vi "Load and Save Data (Burst Shape Data).vi"(0 "VISA resource name":refnum<visa-resource-name>, 1 "Rise Points Values":dbl[](array[numeric])=[0.0, 0.0] format="%.1f", 5 "Destination File":string, 7 "Rise Points(2)":u32=2, 9 "Fall Points(2)":u32=2, 11 "error in (no error)":errorcluster, 12 "Fall Points Values":dbl[](array[numeric])=[0.0, 0.0] format="%.1f") -> (4 "VISA resource name out":refnum<visa-resource-name>, 15 "error out":errorcluster)   [LabVIEW 2018, in "Agilent PSG MXG Series.lvlib"]
doc: "Loads a burst shape file into the signal generators' non-volatile memory(NVWFM). \n\n<B>Note:</B>\nThis VI is only valid in N5172B that installs with <B>Option 653</B> or <B>Option 655</B>, or N5182B that installs with <B>Option 656</B> or <B>Option 657</B>."
uses:
  Agilent PSG MXG Series.lvlib
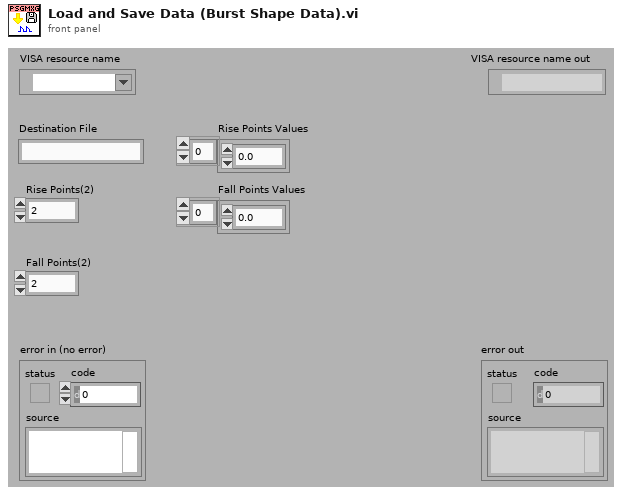
[diagram p1: front panel]
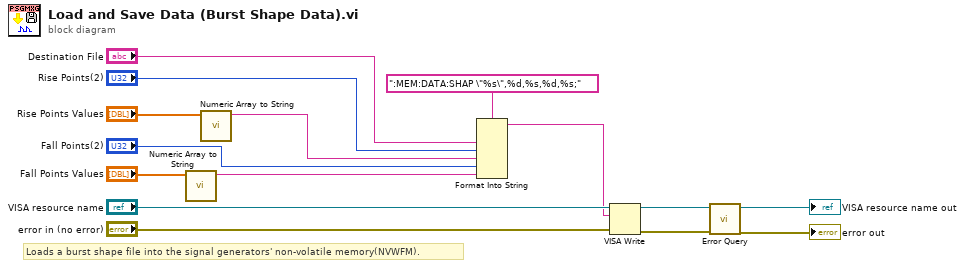
[diagram p0: block diagram]
diagram:
  # "Loads a burst shape file into the signal generators' non-volatile memory(NVWFM)."
  n1 = call "Numeric Array to String.vi"("Numeric Array"="Fall Points Values") -> ("Output String"=w6:string)  [unwired: 10 in]
  n2 = call "Numeric Array to String.vi"("Numeric Array"="Rise Points Values") -> ("Output String"=w4:string)  [unwired: 10 in]
  n3 = Format Into String(format string=":MEM:DATA:SHAP \"%s\",%d,%s,%d,%s;", "Destination File", "Rise Points(2)", w4, "Fall Points(2)", w6) -> (resulting string=w8:string)  [unwired: 2 in, 1 out]
  n4 = VISA Write(VISA resource name="VISA resource name", write buffer=w8, error in (no error)="error in (no error)") -> (VISA resource name out=w15:refnum<visa-resource-name>, error out=w14:errorcluster)  [unwired: 1 out]
  n5 = call "Error Query.vi"("error in (no error)"=w14, "VISA resource name"=w15) -> ("error out"=→"error out":errorcluster, "VISA resource name out"=→"VISA resource name out":refnum<visa-resource-name>)  [unwired: 6 in, 2 out]
